vi "Initialize.vi"(8 "error in (no error)":errorcluster, 10 "Function Enqueuer":refnum<class "Message Enqueuer.lvclass">, 11 "TriggerAction in":refnum<class "TriggerAction Q.lvclass">) -> (0 "error out":errorcluster, 3 "TriggerAction out":refnum<class "TriggerAction Q.lvclass">)   [LabVIEW 2016, in "TriggerAction Q.lvclass"]
uses:
  <userlib>/Common Components/TriggerAction Q/TriggerAction Q/TriggerAction Q.lvclass
  <vilib>/ActorFramework/Message Enqueuer/Message Enqueuer.lvclass
  <userlib>/Common Components/TriggerAction Q/TriggerAction Q/Element Data.ctl
  <userlib>/Common Components/TriggerAction Q/TriggerAction Q/TriggerAction Q.lvclass/TriggerAction Q.ctl
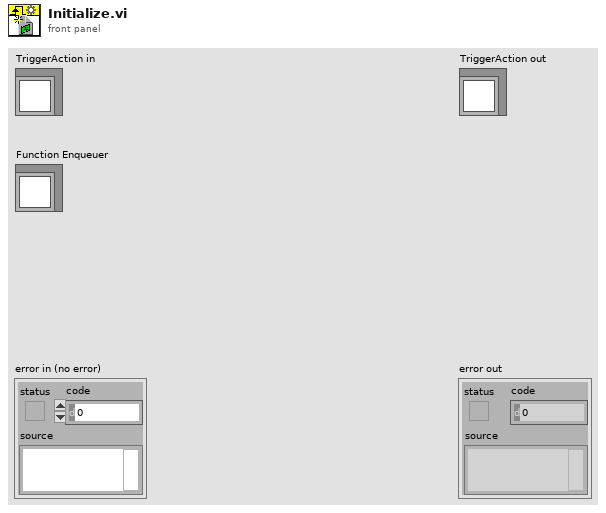
[diagram p1: front panel]
types:
  T1 = typedef "TriggerAction Q.lvclass/Element Data.ctl" = cluster{"Triggers":cluster{"Triggers for Array AND":string[]}[], "Actions":cluster{"Action Name":string, "Action Data":string}[]}
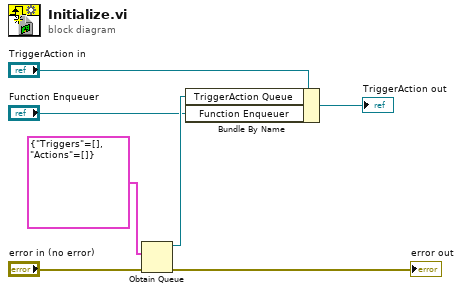
[diagram p0: block diagram]
diagram:
  n1 = Obtain Queue(element data type=T1 {"Triggers"=[], "Actions"=[]} ("Cluster"), error in (no error)="error in (no error)") -> (queue out=w4:refnum<queue>, error out=→"error out":errorcluster)  [unwired: 3 in, 1 out]
  n2 = Bundle By Name(cluster="TriggerAction in", "TriggerAction Queue"=w4, "Function Enqueuer"="Function Enqueuer") -> (→"TriggerAction out":refnum<class "TriggerAction Q.lvclass">)
